vi "Configure Resistance Voltage Source.vi"(0 "VISA resource name":refnum<visa-resource-name>, 1 "Voltage Source Level (0.000000E+0)":dbl format="%.6e", 2 "Manual Range (2.0000000E-2)":dbl=0.02 format="%.7e", 5 "Voltage Source Mode (0: Manual)":i32(ring) items=["Manual", "Auto"], 7 "Enable Voltage Source (F: Disable)":bool, 9 "Voltage Source Range (1.0000000E+2)":dbl=100.0 format="%.7e", 11 "error in (no error)":errorcluster, 12 "Auto Range (1: ON)":i32(ring)=1 items=["OFF", "ON", "ONCE"]) -> (4 "VISA resource name out":refnum<visa-resource-name>, 15 "error out":errorcluster)   [LabVIEW 2019, in "Keithley 6517.lvlib"]
doc: "Controls V-Source and manual auto range, sets V-Source mode, range and level and measurement range for Manual V-source Ohms.\n\n<B>Note:</B>\nThis VI is <B>NOT</B> compatible with model <B>6514</B>."
uses:
  Keithley 6517.lvlib
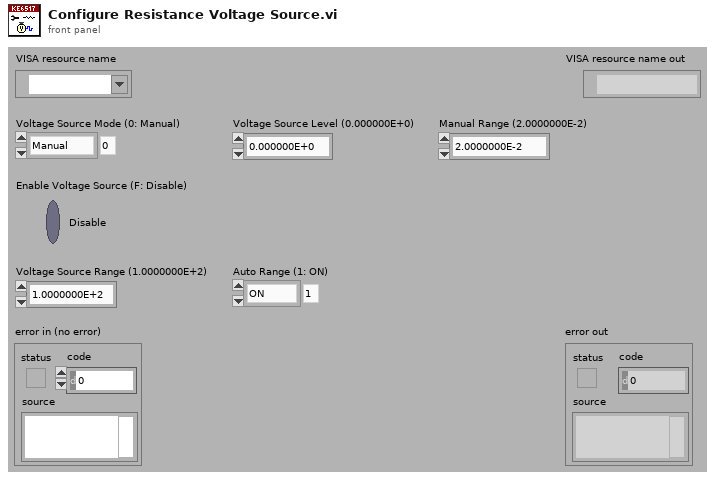
[diagram p1: front panel]
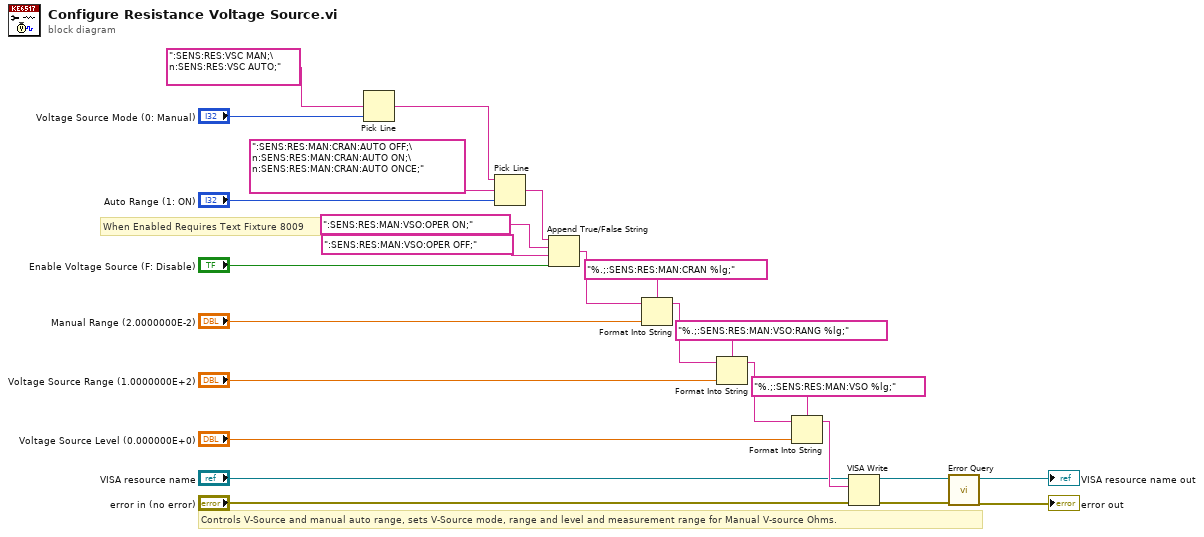
[diagram p0: block diagram]
diagram:
  # "When Enabled Requires Text Fixture 8009"
  # "Controls V-Source and manual auto range, sets V-Source mode, range and level and measurement range for Manual V-source Ohms."
  n1 = Pick Line(multi-line string=":SENS:RES:VSC MAN;\n:SENS:RES:VSC AUTO;", line index="Voltage Source Mode (0: Manual)") -> (output string=w4:string)  [unwired: 1 in]
  n2 = Pick Line(string ("")=w4, multi-line string=":SENS:RES:MAN:CRAN:AUTO OFF;\n:SENS:RES:MAN:CRAN:AUTO ON;\n:SENS:RES:MAN:CRAN:AUTO ONCE;", line index="Auto Range (1: ON)") -> (output string=w1:string)
  n3 = Append True/False String(1:"Enable Voltage Source (F: Disable)", 2:":SENS:RES:MAN:VSO:OPER OFF;", 3:":SENS:RES:MAN:VSO:OPER ON;", 4:w1) -> (0:w22:string)
  n4 = Format Into String(format string="%.;:SENS:RES:MAN:CRAN %lg;", initial string=w22, "Manual Range (2.0000000E-2)") -> (resulting string=w19:string)  [unwired: 1 in, 1 out]
  n5 = Format Into String(format string="%.;:SENS:RES:MAN:VSO:RANG %lg;", initial string=w19, "Voltage Source Range (1.0000000E+2)") -> (resulting string=w16:string)  [unwired: 1 in, 1 out]
  n6 = Format Into String(format string="%.;:SENS:RES:MAN:VSO %lg;", initial string=w16, "Voltage Source Level (0.000000E+0)") -> (resulting string=w13:string)  [unwired: 1 in, 1 out]
  n7 = VISA Write(VISA resource name="VISA resource name", write buffer=w13, error in (no error)="error in (no error)") -> (VISA resource name out=w10:refnum<visa-resource-name>, error out=w9:errorcluster)  [unwired: 1 out]
  n8 = call "Error Query.vi"("error in (no error)"=w9, "VISA resource name"=w10) -> ("error out"=→"error out":errorcluster, "VISA resource name out"=→"VISA resource name out":refnum<visa-resource-name>)  [unwired: 6 in, 2 out]
